vi "To Variant.vi"(8 "error in (no error)":errorcluster, 9 "datatype and defaults":variant, 11 "JSON Datatype in":refnum<class "JSON Datatype.lvclass">) -> (0 "error out":errorcluster, 2 "Variant":variant)   [LabVIEW 2015, in "LVJSON.lvlib" / "JSON Datatype.lvclass"]
uses:
  JSON Datatype.lvclass
  To More Specific Type (Array).vi
  To More Specific Type (Numeric).vi
  JSON Numeric/Read value (Numeric).vi
  To More Specific Type (Boolean).vi
  JSON Boolean/Read value (Boolean).vi
  To More Specific Type (String).vi
  JSON String/Read value (String).vi
  To More Specific Type (Object).vi
  <vilib>/Utility/Data Type/NI_Data Type.lvlib
  JSON Array/JSON Array.lvclass
  JSON Object/JSON Object.lvclass
  JSON Basic Type/JSON Basic Type.lvclass
  JSON String/JSON String.lvclass
  JSON Boolean/JSON Boolean.lvclass
  JSON Numeric/JSON Numeric.lvclass
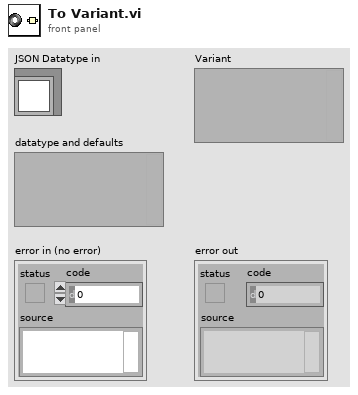
[diagram p1: front panel]
types:
  T1 = typedef "NI_Data Type.lvlib/Data Type.ctl" = enum8{"Invalid Type", "Void", "I8", "I16", "I32", "I64", "U8", "U16", "U32", "U64", "Single Float", "Double Float", "Extended Float", "Single Complex", "Double Complex", "Extended Complex", "Enum U8", "Enum U16", "Enum U32", "Enum U64", "Single Float With Unit", "Double Float With Unit", "Extended Float With Unit", "Single Complex with Unit", "Double Complex with Unit", "Extended Complex with Unit", "Boolean", "String", "Path", "Picture", "Tag", "Array", "Cluster", "Variant", "LV Variant", "Waveform", "Timestamp", "Digital Waveform", "Digital Data", "ExpressData", "Refnum", "External Data", "VI", "Poly VI", "LabVIEW Class Instance", "Fixed Point"}
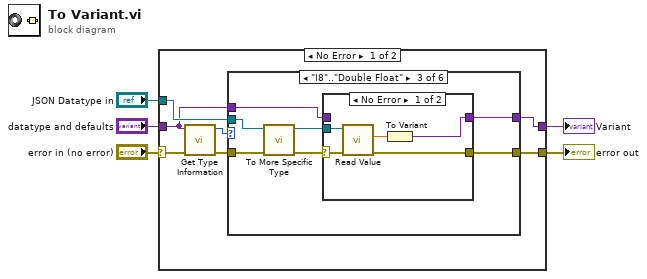
[diagram p0: block diagram]
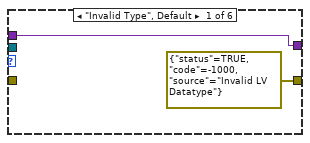
[diagram p2: hidden frame]
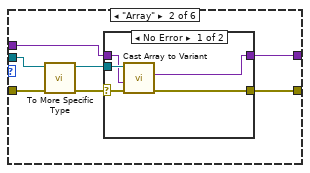
[diagram p3: hidden frame]
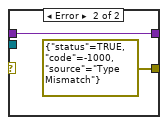
[diagram p4: hidden frame]
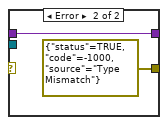
[diagram p5: hidden frame]
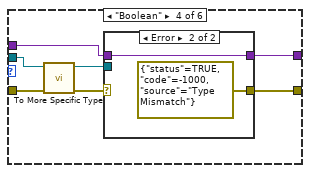
[diagram p6: hidden frame]
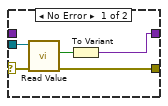
[diagram p7: hidden frame]
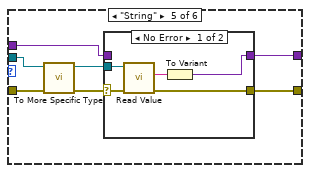
[diagram p8: hidden frame]
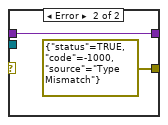
[diagram p9: hidden frame]
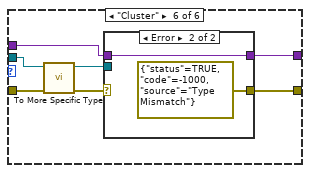
[diagram p10: hidden frame]
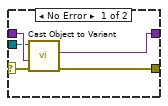
[diagram p11: hidden frame]
diagram:
  n1 = case shown="No Error" "error in (no error)" {
    selector: "error in (no error)" -> [w8 w86]
    tunnel: [w6 w86] -> w4
    tunnel: "JSON Datatype in" -> [w11 _]
    tunnel: "datatype and defaults" -> [w9 w85]
    tunnel: [w10 w85] -> w1
    frame No Error {
      n2 = call <vilib>:"Get Type Information.vi"("error in (no error)"=w8, "Variant"=w9) -> ("error out"=w7:errorcluster, "Type"=w12:T1)  [unwired: 5 in, 3 out]
      n3 = case shown="\"I8\"..\"Double Float\"" w12 {
        tunnel: w11 -> [_ w21 w35 w49 w63 w77]
        tunnel: [w14 w15 w29 w45 w58 w74] -> w10
        tunnel: w9 -> [w14 w17 w33 w46 w57 w76]
        tunnel: w7 -> [_ w20 w34 w48 w62 w73]
        tunnel: [errorcluster {"status"=TRUE, "code"=-1000, "source"="Invalid LV Datatype"} ("error out") w18 w30 w44 w59 w71] -> w6
        frame "Invalid Type", Default {
        }
        frame "Array" {
          n4 = call-poly "To More Specific Type.vi"("error in (no error)"=w20, "JSON Datatype in"=w21) -> ("error out"=w19:errorcluster, "JSON Datatype out"=w16:refnum<class "JSON Array.lvclass">)  [unwired: 8 in]
          n5 = case shown="No Error" w19 {
            selector: w19 -> [w24 _]
            tunnel: [w25 errorcluster {"status"=TRUE, "code"=-1000, "source"="Type Mismatch"} ("error out")] -> w18
            tunnel: [w26 w28] -> w15
            tunnel: w17 -> [w22 w28]
            tunnel: w16 -> [w23 _]
            frame No Error {
              n6 = call "Cast Array to Variant.vi"("error in (no error)"=w24, "datatype and defaults"=w22, "JSON Array in"=w23) -> ("error out"=w25:errorcluster, "Variant"=w26:variant)  [unwired: 7 in]
            }
            frame Error {
            }
          }
        }
        frame "I8".."Double Float" {
          n7 = call-poly "To More Specific Type.vi"("error in (no error)"=w34, "JSON Datatype in"=w35) -> ("error out"=w31:errorcluster, "JSON Numeric out"=w32:refnum<class "JSON Numeric.lvclass">)  [unwired: 8 in]
          n8 = case shown="No Error" w31 {
            selector: w31 -> [w39 _]
            tunnel: w32 -> [w40 _]
            tunnel: [w38 errorcluster {"status"=TRUE, "code"=-1000, "source"="Type Mismatch"} ("error out")] -> w30
            tunnel: [w37 w42] -> w29
            tunnel: w33 -> [_ w42]
            frame No Error {
              n9 = call-poly "Read Value.vi"("error in (no error)"=w39, "JSON String in"=w40) -> ("error out"=w38:errorcluster, "value"=w36:dbl)  [unwired: 7 in, 1 out]
              n10 = To Variant(anything=w36) -> (Variant=w37:variant)
            }
            frame Error {
            }
          }
        }
        frame "Boolean" {
          n11 = call-poly "To More Specific Type.vi"("error in (no error)"=w48, "JSON Datatype in"=w49) -> ("error out"=w43:errorcluster, "JSON Datatype out"=w47:refnum<class "JSON Boolean.lvclass">)  [unwired: 8 in]
          n12 = case shown="Error" w43 {
            selector: w43 -> [w53 _]
            tunnel: w47 -> [w54 _]
            tunnel: [w52 errorcluster {"status"=TRUE, "code"=-1000, "source"="Type Mismatch"} ("error out")] -> w44
            tunnel: [w51 w56] -> w45
            tunnel: w46 -> [_ w56]
            frame No Error {
              n13 = call-poly "Read Value.vi"("error in (no error)"=w53, "JSON String in"=w54) -> ("error out"=w52:errorcluster, "value"=w50:bool)  [unwired: 7 in, 1 out]
              n14 = To Variant(anything=w50) -> (Variant=w51:variant)
            }
            frame Error {
            }
          }
        }
        frame "String" {
          n15 = call-poly "To More Specific Type.vi"("error in (no error)"=w62, "JSON Datatype in"=w63) -> ("error out"=w60:errorcluster, "JSON Datatype out"=w61:refnum<class "JSON String.lvclass">)  [unwired: 8 in]
          n16 = case shown="No Error" w60 {
            selector: w60 -> [w67 _]
            tunnel: w61 -> [w68 _]
            tunnel: [w66 errorcluster {"status"=TRUE, "code"=-1000, "source"="Type Mismatch"} ("error out")] -> w59
            tunnel: [w65 w70] -> w58
            tunnel: w57 -> [_ w70]
            frame No Error {
              n17 = call-poly "Read Value.vi"("error in (no error)"=w67, "JSON String in"=w68) -> ("error out"=w66:errorcluster, "value"=w64:string)  [unwired: 7 in, 1 out]
              n18 = To Variant(anything=w64) -> (Variant=w65:variant)
            }
            frame Error {
            }
          }
        }
        frame "Cluster" {
          n19 = call-poly "To More Specific Type.vi"("error in (no error)"=w73, "JSON Datatype in"=w77) -> ("error out"=w72:errorcluster, "JSON Datatype out"=w75:refnum<class "JSON Object.lvclass">)  [unwired: 8 in]
          n20 = case shown="Error" w72 {
            selector: w72 -> [w79 _]
            tunnel: w76 -> [w82 w84]
            tunnel: w75 -> [w81 _]
            tunnel: [w80 w84] -> w74
            tunnel: [w78 errorcluster {"status"=TRUE, "code"=-1000, "source"="Type Mismatch"} ("error out")] -> w71
            frame No Error {
              n21 = call "Cast Object to Variant.vi"("error in (no error)"=w79, "datatype and defaults"=w82, "JSON Object in"=w81) -> ("error out"=w78:errorcluster, "Variant"=w80:variant)  [unwired: 7 in]
            }
            frame Error {
            }
          }
        }
      }
    }
    frame Error {
    }
  }
  "error out" <- w4
  "Variant" <- w1
